vi "Drive Straight (SubVI).vi"(6 "Slow Down time":u32, 7 "Drive Time":u32, 9 "AutoY":dbl, 11 "DriveMotorRefNum":string="RobotDrive") -> (3 "String":string)   [LabVIEW 2017]
uses:
  <vilib>/Rock Robotics/WPI/SafetyOutput/WPI_SafetyOutputConfigMenu.ctl
  Robot Global Data.vi
  <vilib>/Rock Robotics/WPI/Utilities/WPI_GetSetVariantRefNum.vi
  <vilib>/Rock Robotics/WPI/RobotDrive/WPI_RobotDriveArcadeDrive_Standard(NoSaturation).vi
  <vilib>/Rock Robotics/WPI/RobotDrive/WPI_RobotDriveSafetyCheck.vi
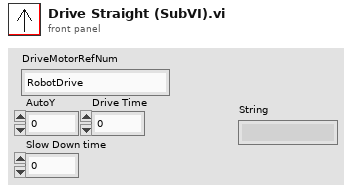
[diagram p1: front panel]
types:
  T1 = typedef "WPI_SafetyOutputConfigMenu.ctl" = enum16{"Enable", "Disable"}
  T2 = typedef "WPI_RobotDriveDevRef.ctl" = cluster{"DevStatus":errorcluster, "Motors[]":T3[], "Square Inputs":bool, "Max Output":dbl}
  T3 = typedef "WPI_MotorControlDeviceRef.ctl" = cluster{"DeviceStatus":errorcluster, "Type":T4, "PWM":cluster{"PWM Channel":T5, "DeadBand":T6}, "CAN":cluster{"Device Number":u8, "SetOutput VI Ref":variant, "GetOutput VI Ref":variant, "Enable VI Ref":variant, "Disable VI Ref":variant, "Data":variant}, "Invert":bool, "DIO PWM":cluster{"PWM \"Enable\" Channel":T5, "DIOChannel":T7, "PWM Rate":dbl}}
  T4 = typedef "WPI_MotorControlType.ctl" = enum16{"PWM", "CAN", "DIO PWM"}
  T5 = typedef "FPGA_DIOPWMChannel.ctl" = enum8{"PWM 0", "PWM 1", "PWM 2", "PWM 3", "PWM 4", "PWM 5", "PWM 6", "PWM 7", "PWM 8", "PWM 9", "PWM MXP 0", "PWM MXP 1", "PWM MXP 2", "PWM MXP 3", "PWM MXP 4", "PWM MXP 5", "PWM MXP 6", "PWM MXP 7", "PWM MXP 8", "PWM MXP 9", "Invalid"}
  T6 = typedef "WPI_PWMDeadband.ctl" = cluster{"Name":string, "maxPositivePwm":i32, "minPositivePwm":i32, "centerPwm":i32, "maxNegativePwm":i32, "minNegativePwm":i32, "angularRange":u16}
  T7 = typedef "FPGA_DIOChannel.ctl" = enum8{"DIO 0", "DIO 1", "DIO 2", "DIO 3", "DIO 4", "DIO 5", "DIO 6", "DIO 7", "DIO 8", "DIO 9", "DIO MXP 0", "DIO MXP 1", "DIO MXP 2", "DIO MXP 3", "DIO MXP 4", "DIO MXP 5", "DIO MXP 6", "DIO MXP 7", "DIO MXP 8", "DIO MXP 9", "DIO MXP 10", "DIO MXP 11", "DIO MXP 12", "DIO MXP 13", "DIO MXP 14", "DIO MXP 15", "SPI Port CS1", "SPI Port CS2", "SPI Port CS3", "SPI Port MISO", "SPI Port MOSI", "Invalid"}
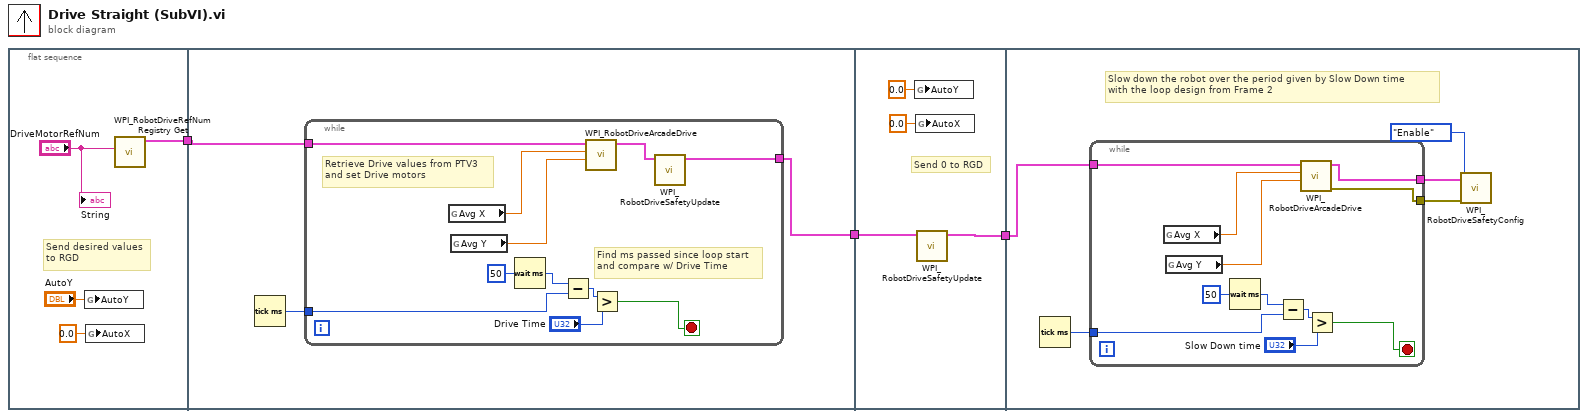
[diagram p0: block diagram]
diagram:
  n1 = flat-sequence {
    tunnel: [w7] -> w3
    tunnel: w3 -> [w9]
    tunnel: [w8] -> w2
    tunnel: [w24] -> w1
    tunnel: w2 -> [w25]
    tunnel: w1 -> [w29]
    frame #0 {
      # "Send desired values\nto RGD"
      n2 = global write "Robot Global Data.vi" "AutoY"("AutoY") -> ()
      n3 = global write "Robot Global Data.vi" "AutoX"(0.0 ("AutoX")) -> ()
      n4 = call <vilib>:"WPI_RobotDriveRefNum Registry Get.vi"("refnum name"="DriveMotorRefNum") -> ("RobotDriveDevRef"=w7:T2)  [unwired: 9 in, 1 out]
      "String" <- "DriveMotorRefNum"
    }
    frame #1 {
      n5 = Tick Count (ms)() -> (millisecond timer value=w10:u32)
      n6 = while {
        tunnel: w9 -> [w19]
        tunnel: [w11] -> w8
        tunnel: w10 -> [w16]
        stop <- w17 stop-if-true
        # "Retrieve Drive values from PTV3\nand set Drive motors"
        # "Find ms passed since loop start\nand compare w/ Drive Time"
        n7 = global read "Robot Global Data.vi" "Avg X"() -> (w21:dbl)
        n8 = global read "Robot Global Data.vi" "Avg Y"() -> (w20:dbl)
        n9 = Wait (ms)(milliseconds to wait=u32 50) -> (millisecond timer value=w15:u32)
        n10 = Subtract(x=w15, y=w16) -> (x-y=w14:u32)
        n11 = call-poly <vilib>:"WPI_RobotDriveArcadeDrive.vi"("Y axis value"=w20, "X axis value"=w21, "RobotDriveDevRef"=w19) -> ("RobotDriveDevRef"=w13:T2)  [unwired: 6 in, 2 out]
        n12 = Greater?(x=w14, y="Drive Time") -> (0:w17:bool)
        n13 = call <vilib>:"WPI_RobotDriveSafetyUpdate.vi"("RobotDriveDevRef"=w13) -> ("RobotDriveDevRef"=w11:T2)  [unwired: 1 in, 9 out]
      }
    }
    frame #2 {
      # "Send 0 to RGD"
      n14 = global write "Robot Global Data.vi" "AutoY"(0.0 ("AutoY")) -> ()
      n15 = global write "Robot Global Data.vi" "AutoX"(0.0 ("AutoX")) -> ()
      n16 = call <vilib>:"WPI_RobotDriveSafetyUpdate.vi"("RobotDriveDevRef"=w25) -> ("RobotDriveDevRef"=w24:T2)  [unwired: 1 in, 9 out]
    }
    frame #3 {
      # "Slow down the robot over the period given by Slow Down time\nwith the loop design from Frame 2"
      n17 = Tick Count (ms)() -> (millisecond timer value=w30:u32)
      n18 = while {
        tunnel: w29 -> [w39]
        tunnel: [w36] -> w28
        tunnel: w30 -> [w35]
        tunnel: [w33] -> w27
        stop <- w37 stop-if-true
        n19 = global read "Robot Global Data.vi" "Avg X"() -> (w41:dbl)
        n20 = global read "Robot Global Data.vi" "Avg Y"() -> (w40:dbl)
        n21 = Wait (ms)(milliseconds to wait=u32 50) -> (millisecond timer value=w34:u32)
        n22 = Subtract(x=w34, y=w35) -> (x-y=w32:u32)
        n23 = call-poly <vilib>:"WPI_RobotDriveArcadeDrive.vi"("Y axis value"=w40, "X axis value"=w41, "RobotDriveDevRef"=w39) -> ("error out"=w33:errorcluster, "RobotDriveDevRef"=w36:T2)  [unwired: 6 in, 1 out]
        n24 = Greater?(x=w32, y="Slow Down time") -> (0:w37:bool)
      }
      n25 = call <vilib>:"WPI_RobotDriveSafetyConfig.vi"("error in (no error)"=w27, "mode"=WPI_SafetyOutputConfigMenu."Enable", "RobotDriveDevRef"=w28) -> ()  [unwired: 7 in, 2 out]
    }
  }
